vi "file log variable.vi"(0 "memory usage":dbl, 1 "file name":string, 2 "X stage position":dbl, 3 "Y stage position":dbl, 4 "slice plane":dbl, 5 "error in":errorcluster, 6 "image plane":dbl, 7 "time":string, 8 "Item":T2=enum."X stage", 9 "Disk full space":dbl, 11 "Disk free space":dbl) -> (14 "First element":T1, 19 "error out":errorcluster)   [LabVIEW 2018]
uses:
  Controls/file variable action.ctl
  Controls/file log.ctl
  Controls/FGV Actions.ctl
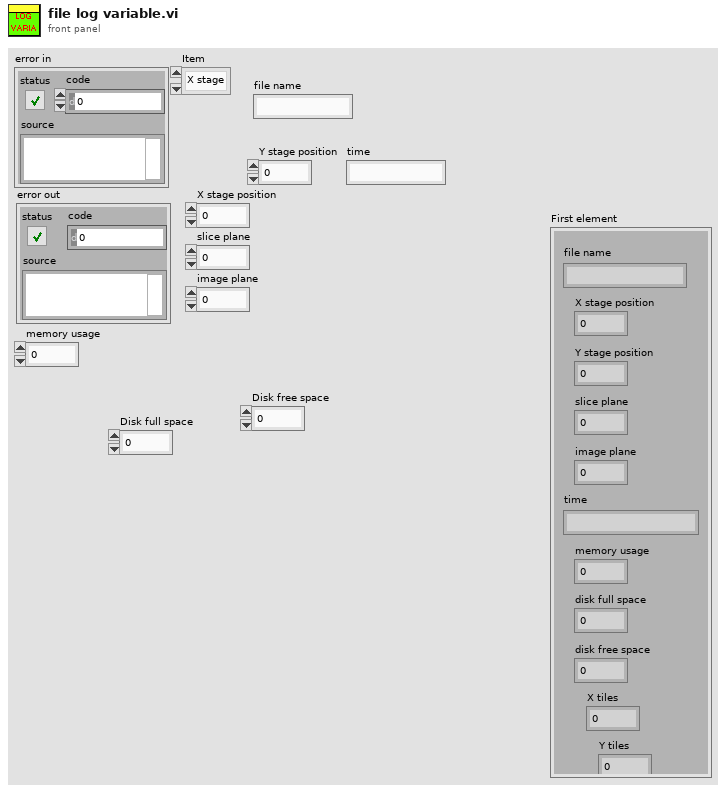
[diagram p1: front panel]
types:
  T1 = typedef "file log.ctl" = cluster{"file name":string, "X stage position":dbl, "Y stage position":dbl, "slice plane":dbl, "image plane":dbl, "time":string, "memory usage":dbl, "disk free space":dbl, "disk full space":dbl, "X tiles":u32, "Y tiles":u32}
  T2 = typedef "file variable action.ctl" = enum16{"File name", "X stage", "Y stage", "Slice plane", "Image plane", "time", "output", "Init", "Memory Usage", "Disk full Space", "Disk free space", "Y tiles", "X tiles"}
  T3 = typedef "FGV Actions.ctl" = enum16{"Init", "Set", "Get", "Clear"}
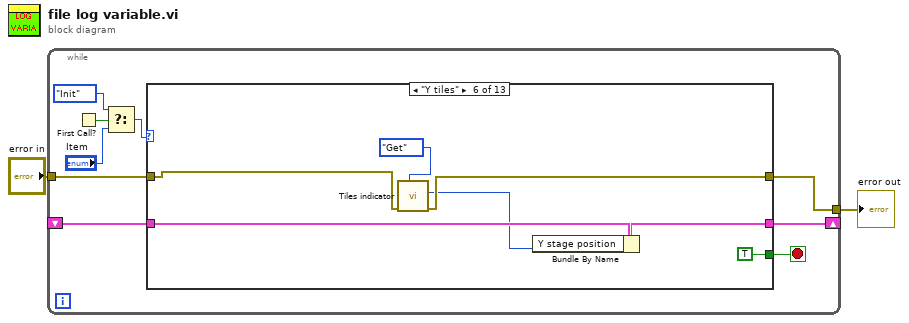
[diagram p0: block diagram]
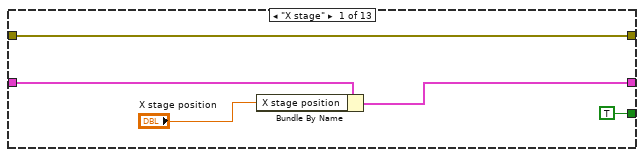
[diagram p2: hidden frame]
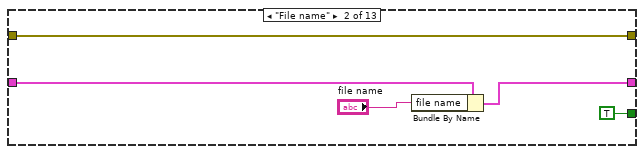
[diagram p3: hidden frame]
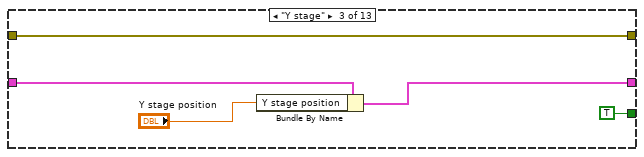
[diagram p4: hidden frame]
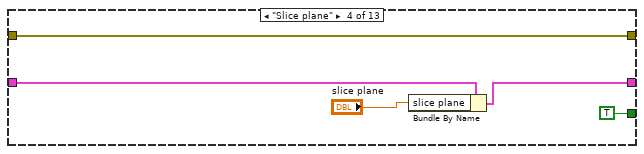
[diagram p5: hidden frame]
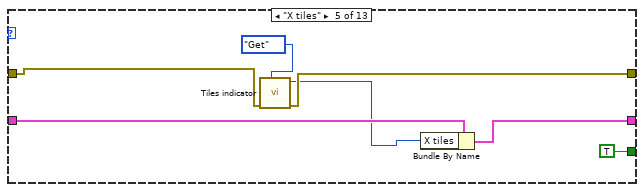
[diagram p6: hidden frame]
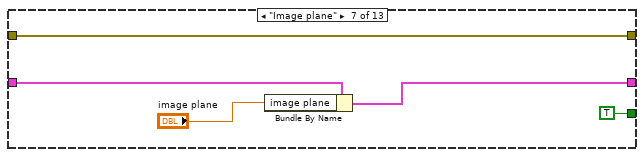
[diagram p7: hidden frame]
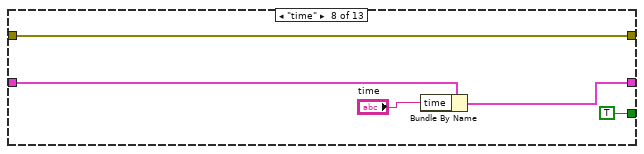
[diagram p8: hidden frame]
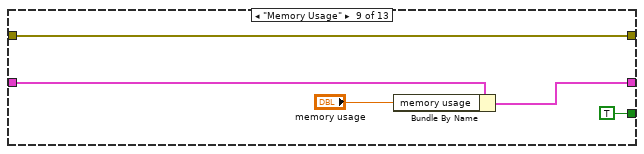
[diagram p9: hidden frame]
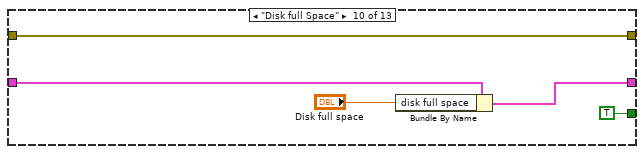
[diagram p10: hidden frame]
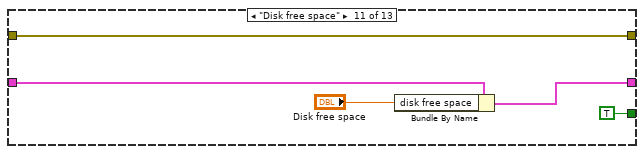
[diagram p11: hidden frame]
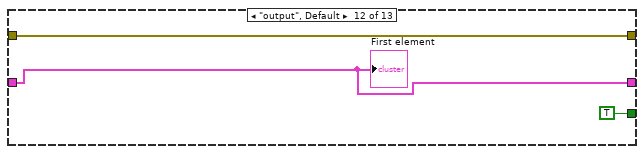
[diagram p12: hidden frame]
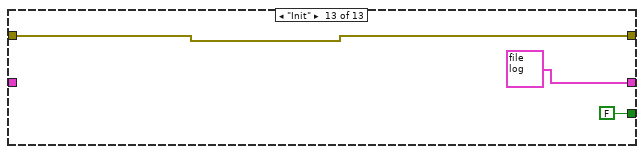
[diagram p13: hidden frame]
diagram:
  n1 = while {
    shift-right: [w10] -> _
    shift-left: _ -> [w11]
    tunnel: "error in" -> [w9]
    tunnel: [w8] -> w1
    stop <- w7 stop-if-true
    n2 = First Call?() -> (First Call?: T/F=w5:bool)
    n3 = Select(t=file_variable_action."Init", s=w5, f="Item") -> (s? t:f=w3:T2)
    n4 = case shown="\"Y tiles\"" w3 {
      tunnel: w11 -> [w13 w18 w23 w28 w37 w44 w47 w52 w57 w62 w67 w71 _]
      tunnel: [w12 w17 w22 w27 w36 w43 w46 w51 w56 w61 w66 w71 T1 {"file name"="", "X stage position"=0.0, "Y stage position"=0.0, "slice plane"=0.0, "image plane"=0.0, "time"="", "memory usage"=0.0, "disk free space"=0.0, "disk full space"=0.0, "X tiles"=0, "Y tiles"=0} ("File Log Array")] -> w10
      tunnel: [w15 w20 w25 w30 w34 w41 w49 w54 w60 w65 w70 w73 w74] -> w8
      tunnel: w9 -> [w15 w20 w25 w30 w35 w42 w49 w54 w60 w65 w70 w73 w74]
      tunnel: [TRUE TRUE TRUE TRUE TRUE TRUE TRUE TRUE TRUE TRUE TRUE TRUE FALSE] -> w7
      frame "X stage" {
        n5 = Bundle By Name(cluster=w13, "X stage position"="X stage position") -> (w12:T1)
      }
      frame "File name" {
        n6 = Bundle By Name(cluster=w18, "file name"="file name") -> (w17:T1)
      }
      frame "Y stage" {
        n7 = Bundle By Name(cluster=w23, "Y stage position"="Y stage position") -> (w22:T1)
      }
      frame "Slice plane" {
        n8 = Bundle By Name(cluster=w28, "slice plane"="slice plane") -> (w27:T1)
      }
      frame "X tiles" {
        n9 = call "Tiles indicator.vi"("Actions"=FGV_Actions."Get", "Error In"=w35) -> ("Error Out"=w34:errorcluster, "# X tiles"=w32:u32)  [unwired: 6 in, 2 out]
        n10 = Bundle By Name(cluster=w37, "X tiles"=w32) -> (w36:T1)
      }
      frame "Y tiles" {
        n11 = call "Tiles indicator.vi"("Actions"=FGV_Actions."Get", "Error In"=w42) -> ("Error Out"=w41:errorcluster, "# Y tiles"=w39:u32)  [unwired: 6 in, 2 out]
        n12 = Bundle By Name(cluster=w44, "Y stage position"=w39) -> (w43:T1)
      }
      frame "Image plane" {
        n13 = Bundle By Name(cluster=w47, "image plane"="image plane") -> (w46:T1)
      }
      frame "time" {
        n14 = Bundle By Name(cluster=w52, "time"="time") -> (w51:T1)
      }
      frame "Memory Usage" {
        n15 = Bundle By Name(cluster=w57, "memory usage"="memory usage") -> (w56:T1)
      }
      frame "Disk full Space" {
        n16 = Bundle By Name(cluster=w62, "disk full space"="Disk full space") -> (w61:T1)
      }
      frame "Disk free space" {
        n17 = Bundle By Name(cluster=w67, "disk free space"="Disk free space") -> (w66:T1)
      }
      frame "output", Default {
        "First element" <- w71
      }
      frame "Init" {
      }
    }
  }
  "error out" <- w1
